vi "recipeScript tempEventCode.vi"(7 "type":enum16{"init", "write", "read"}(ring), 8 "error in (no error)":errorcluster, 10 "scriptPythonCode in":string, 11 "eventProcess in":string[][](array[string])) -> (0 "error out":errorcluster, 2 "scriptPythonCode out":string, 3 "eventProcess out":string[][](array[string]))   [LabVIEW 2018]
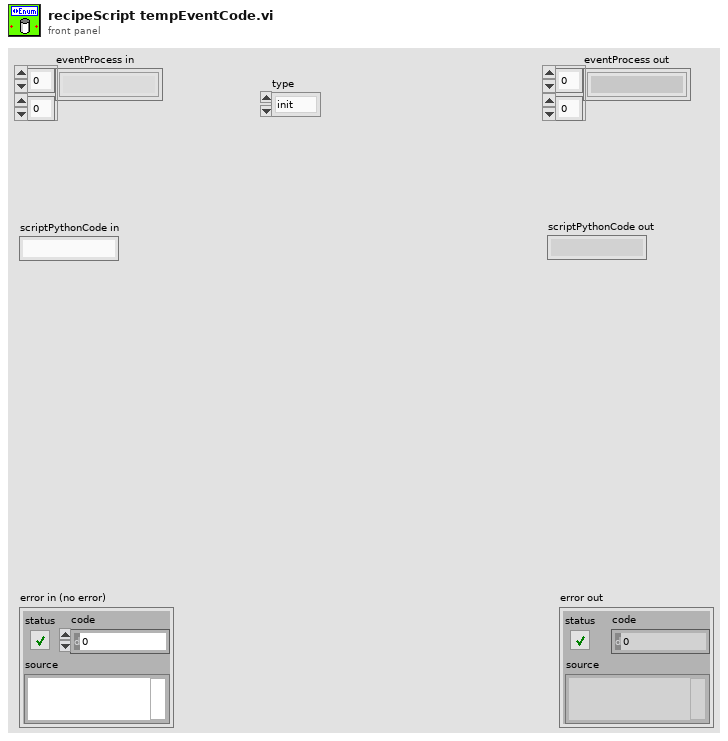
[diagram p1: front panel]
types:
  T1 = cluster{"eventProcess":string[][], "scriptPythonCode":string}
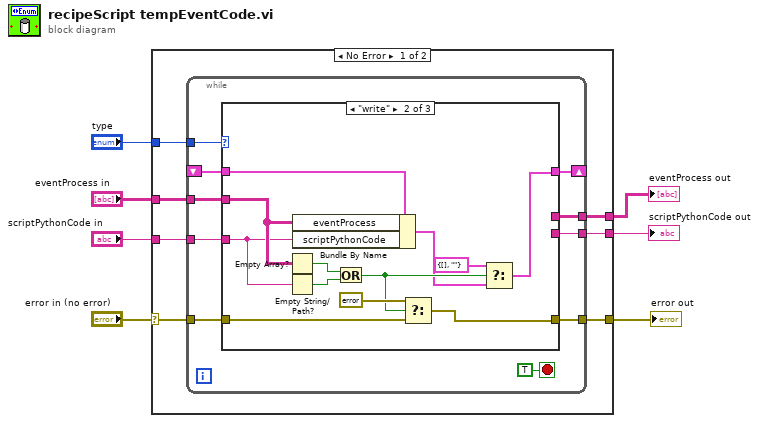
[diagram p0: block diagram]
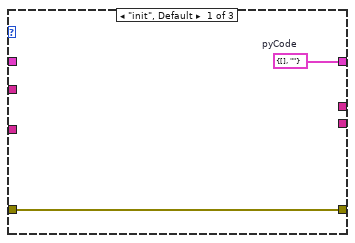
[diagram p2: hidden frame]
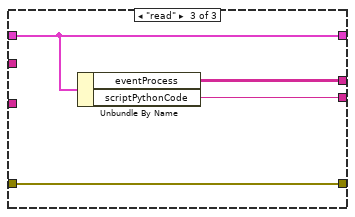
[diagram p3: hidden frame]
diagram:
  n1 = case shown="No Error" "error in (no error)" {
    selector: "error in (no error)" -> [w8 w43]
    tunnel: "type" -> [w14 _]
    tunnel: "eventProcess in" -> [w13 _]
    tunnel: "scriptPythonCode in" -> [w12 _]
    tunnel: [w11 _] -> w4
    tunnel: [w10 _] -> w3
    tunnel: [w9 w43] -> w2
    frame No Error {
      n2 = while {
        tunnel: w14 -> [w24]
        shift-right: [w23] -> _
        shift-left: _ -> [w22]
        tunnel: w13 -> [w21]
        tunnel: w12 -> [w20]
        tunnel: [w18] -> w11
        tunnel: [w17] -> w10
        tunnel: w8 -> [w16]
        tunnel: [w15] -> w9
        stop <- TRUE stop-if-true
        n3 = case shown="\"write\"" w24 {
          tunnel: [w26 w27 w42] -> w23
          tunnel: w22 -> [_ w38 w42]
          tunnel: w21 -> [_ w37 _]
          tunnel: w20 -> [_ w36 _]
          tunnel: [_ _ w41] -> w18
          tunnel: [_ _ w40] -> w17
          tunnel: w16 -> [w25 w33 w39]
          tunnel: [w25 w32 w39] -> w15
          frame "init", Default {
            w26 = T1 {"eventProcess"=[], "scriptPythonCode"=""}  # pyCode
          }
          frame "write" {
            n4 = Empty Array?(array=w37) -> (empty?=w35:bool)
            n5 = Empty String/Path?(string/path=w36) -> (empty?=w34:bool)
            n6 = Bundle By Name(cluster=w38, "eventProcess"=w37, "scriptPythonCode"=w36) -> (w28:T1)
            n7 = Or(x=w35, y=w34) -> (x .or. y?=w30:bool)
            n8 = Select(t=errorcluster {"status"=TRUE, "code"=6012, "source"="Unable to write the script , it's empty."}, s=w30, f=w33) -> (s? t:f=w32:errorcluster)
            n9 = Select(t=T1 {"eventProcess"=[], "scriptPythonCode"=""} ("output cluster"), s=w30, f=w28) -> (s? t:f=w27:T1)
          }
          frame "read" {
            n10 = Unbundle By Name(w42) -> ("eventProcess"=w41:string[][], "scriptPythonCode"=w40:string)
          }
        }
      }
    }
    frame Error {
    }
  }
  "eventProcess out" <- w4
  "scriptPythonCode out" <- w3
  "error out" <- w2
